vi "Analyze.vi"(0 "Analyze SHG-AK in":refnum<class "Analyze SHG-AK.lvclass">, 1 "Create Overlay?":bool, 5 "Image in":T1, 7 "Parameters":variant, 9 "Results in":variant, 11 "error in (no error)":errorcluster) -> (4 "Analyze SHG-AK out":refnum<class "Analyze SHG-AK.lvclass">, 6 "Image out":T1, 8 "Parameters out":variant, 10 "Results":variant, 15 "error out":errorcluster)   [LabVIEW 2014, in "Analyze.lvlib" / "Analyze SHG-AK.lvclass"]
uses:
  Analyze SHG-AK.lvclass
  <vilib>/vision/Image Controls.llb/IMAQ Image.ctl
  Analyze BaseClass/Analyze BaseClass.lvclass
  <vilib>/vision/NI_Vision_Development_Module.lvlib
  XDisplay/POLARIS IMAQ Display.xctl
  <vilib>/Analysis/NI_AALPro.lvlib
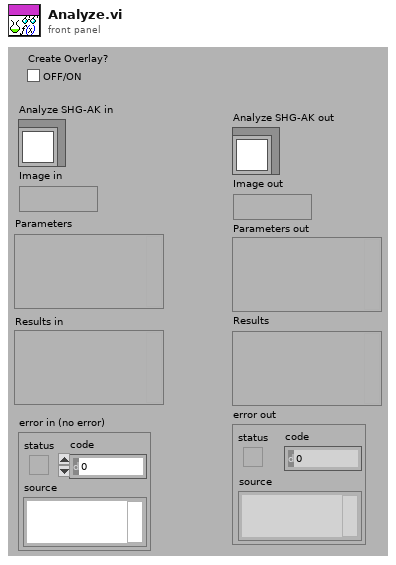
[diagram p1: front panel]
types:
  T1 = typedef "IMAQ Image.ctl" = refnum<image>
  T2 = typedef "ROI Descriptor" = cluster{"Global Rectangle":i32[], "Contours":cluster{"ID":enum32{"External", "Internal"}, "Type":u32, "Coordinates":i32[]}[]}
  T3 = cluster{"Desired Font (Application)":enum16{"User-specified Font", "Application Font", "System Font", "Dialog Font"}, "[User-specified Font]":cluster{"Font Name":string, "Size":i16, "Strikeout?":bool, "Italic?":bool, "Underline?":bool, "Outline?":bool, "Shadow?":bool, "Bold?":bool, "Rotation Angle":dbl}, "Horizontal Alignment":i16, "Vertical Alignment":i16}
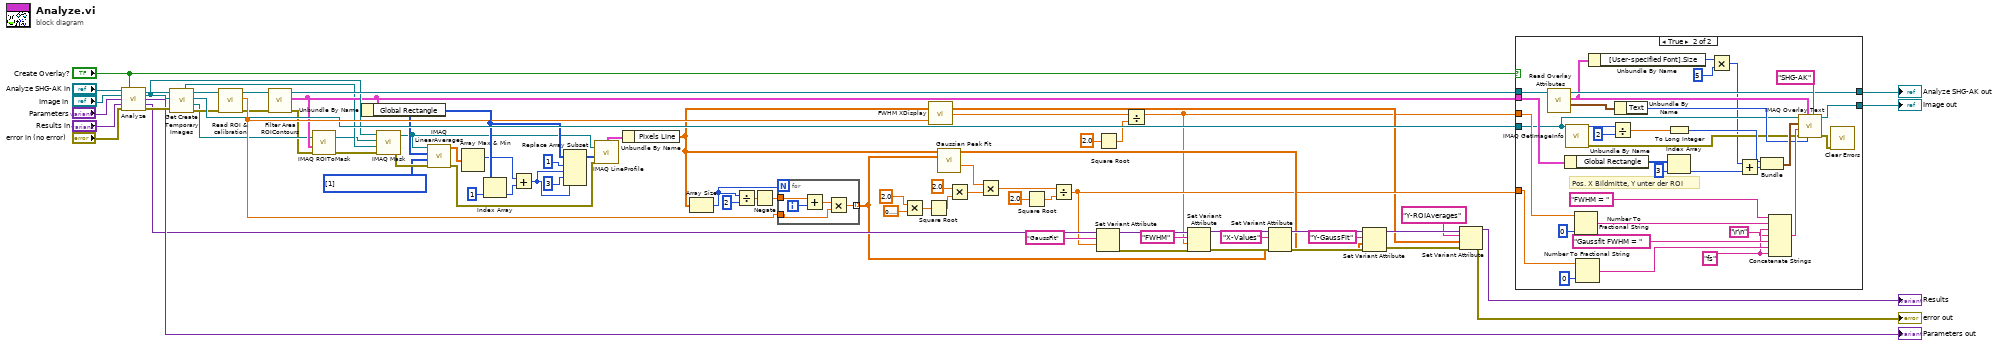
[diagram p0: block diagram]
diagram:
  w13 = i32[] [1] items=["X Axis Averages", "Y Axis Averages", "X + Y Axis Averages", "X - Y Axis Averages"] ("Averages")
  n1 = call-parent "Analyze.vi"("Analyze BaseClass in"="Analyze SHG-AK in", "Create Overlay?"="Create Overlay?", "Image in"="Image in", "Parameters"="Parameters", "Results in"="Results in", "error in (no error)"="error in (no error)") -> ("Analyze BaseClass out"=w72:refnum<class "Analyze SHG-AK.lvclass">, "Image out"=w30:T1, "Parameters out"=→"Parameters out":variant, "Results"=w54:variant, "error out"=w71:errorcluster)  [unwired: 5 in]
  n2 = call-dynamic "Get Create Temporary Images.vi"("error in (no error)"=w71, "Image in"=w30, "Analyze BaseClass in"=w72) -> ("error out"=w22:errorcluster, "image mask"=w21:T1, "work image"=w34:T1, "Analyze BaseClass out"=w23:refnum<class "Analyze SHG-AK.lvclass">, "masked image"=w20:T1)  [unwired: 4 in]
  n3 = call-dynamic "Read ROI & calibration.vi"("error in (no error)"=w22, "Analyze BaseClass in"=w23) -> ("error out"=w16:errorcluster, "calibration mm/px"=w58:dbl, "Analyze BaseClass out"=w17:refnum<class "Analyze SHG-AK.lvclass">)  [unwired: 6 in, 1 out]
  n4 = call-dynamic "Filter Area ROIContours.vi"("error in (no error)"=w16, "Analyze BaseClass in"=w17) -> ("error out"=w15:errorcluster, "ROI of Area type"=w29:T2, "Analyze BaseClass out"=w38:refnum<class "Analyze SHG-AK.lvclass">)  [unwired: 7 in]
  n5 = call "IMAQ ROIToMask"("error in (no error)"=w15, "ROI Descriptor"=w29, "Image"=w21) -> ("error out"=w19:errorcluster, "Image Out"=w18:T1)  [unwired: 3 in, 1 out]
  n6 = Unbundle By Name(w29) -> ("Global Rectangle"=w9:i32[])
  n7 = call "IMAQ Mask"("error in (no error)"=w19, "Image Dst"=w20, "Image Mask"=w18, "Image Src"=w30) -> ("error out"=w14:errorcluster, "Image Dst Out"=w4:T1)  [unwired: 1 in]
  n8 = call "IMAQ LinearAverages"("error in (no error)"=w14, "Averages"=w13, "Optional Rectangle"=w9, "Image Src"=w4) -> ("error out"=w2:errorcluster, "Y Axis Averages"=w12:sgl[])  [unwired: 3 in, 3 out]
  n9 = Array Max & Min(array=w12) -> (max index (indices)=w6:i32)  [unwired: 3 out]
  n10 = Index Array(array=w9, index=1) -> (element=w7:i32)
  n11 = Add(x=w6, y=w7) -> (x+y=w5:i32)
  n12 = Replace Array Subset(array=w9, new element #1=w5, index #1=1 ("index"), new element #2=w5, index #2=3 ("index")) -> (w3:i32[])
  n13 = call "IMAQ LineProfile"("error in (no error)"=w2, "Line Coordinates"=w3, "Image"=w4) -> ("Line Graph"=w1:cluster{"x0":sgl, "dx":sgl, "Pixels Line":sgl[]})  [unwired: 2 in, 3 out]
  n14 = Unbundle By Name(w1) -> ("Pixels Line"=w28:sgl[])
  n15 = Array Size(array=w28) -> (size(s)=w57:i32)
  n16 = Divide(x=w57, y=2) -> (x/y=w60:dbl)
  n17 = Negate(x=w60) -> (-x=w56:dbl)
  n18 = for {
    N: w57 -> [_]
    tunnel: w56 -> [w81]
    tunnel: [w79] -> w47 mode=indexing
    tunnel: w58 -> [w78]
    i -> [w82]
    n19 = Add(x=w81, y=w82) -> (x+y=w80:dbl)
    n20 = Multiply(x=w80, y=w78) -> (x*y=w79:dbl)
  }
  n21 = Multiply(x=2.0 ("y"), y=0.6931471805599453) -> (x*y=w63:dbl)
  n22 = Square Root(x=w63) -> (sqrt(x)=w64:dbl)
  n23 = call "FWHM XDisplay.vi"("calibration"=w58, "array"=w28) -> ("FHWM"=w25:dbl)
  n24 = call <vilib>:"Gaussian Peak Fit.vi"("Y"=w28, "X"=w47) -> ("Best Gaussian Fit"=w42:dbl[], "standard deviation"=w70:dbl)  [unwired: 7 in, 5 out]
  n25 = Multiply(x=2.0 ("y"), y=w64) -> (x*y=w65:dbl)
  n26 = Multiply(x=w70, y=w65) -> (x*y=w68:dbl)
  n27 = Square Root(x=2.0) -> (sqrt(x)=w67:dbl)
  n28 = Divide(x=w68, y=w67) -> (x/y=w36:dbl)
  n29 = Set Variant Attribute(Variant=w54, name="GaussFit", value=w36) -> (Variant out=w52:variant, error out=w50:errorcluster)  [unwired: 1 in, 1 out]
  n30 = Square Root(x=2.0) -> (sqrt(x)=w26:dbl)
  n31 = Divide(x=w25, y=w26) -> (x/y=w24:dbl)
  n32 = Set Variant Attribute(Variant=w52, name="FWHM", value=w24, error in=w50) -> (Variant out=w48:variant, error out=w49:errorcluster)  [unwired: 1 out]
  n33 = Set Variant Attribute(Variant=w48, name="X-Values", value=w47, error in=w49) -> (Variant out=w44:variant, error out=w45:errorcluster)  [unwired: 1 out]
  n34 = Set Variant Attribute(Variant=w44, name="Y-GaussFit", value=w42, error in=w45) -> (Variant out=w41:variant, error out=w40:errorcluster)  [unwired: 1 out]
  n35 = Set Variant Attribute(Variant=w41, name="Y-ROIAverages", value=w28, error in=w40) -> (Variant out=→"Results":variant, error out=→"error out":errorcluster)  [unwired: 1 out]
  n36 = case shown="True" "Create Overlay?" {
    tunnel: w38 -> [w84 w113]
    tunnel: w36 -> [_ w98]
    tunnel: w24 -> [_ w102]
    tunnel: [w84 w112] -> w35
    tunnel: w29 -> [_ w115]
    tunnel: w34 -> [w83 w96]
    tunnel: [w83 w95] -> w33
    frame False {
    }
    frame True {
      w87 = "fs" ("string")
      # "Pos. X Bildmitte, Y unter der ROI"
      n37 = call-dynamic "Read Overlay Attributes.vi"("Analyze BaseClass in"=w113) -> ("Overlay colors"=w111:cluster{"Border":u32, "Text":u32}, "Font, Size & Style"=w92:T3, "Analyze BaseClass out"=w112:refnum<class "Analyze SHG-AK.lvclass">)  [unwired: 6 in, 2 out]
      n38 = Unbundle By Name(w115) -> ("Global Rectangle"=w118:i32[])
      n39 = call "IMAQ GetImageInfo"("Image"=w96) -> ("error out"=w94:errorcluster, "X Resolution"=w109:i32)  [unwired: 3 in, 6 out]
      n40 = Number To Fractional String(number=w102, precision (6)=i16 0) -> (F-format string=w88:string)  [unwired: 2 in]
      n41 = Number To Fractional String(number=w98, precision (6)=i16 0) -> (F-format string=w97:string)  [unwired: 2 in]
      n42 = Unbundle By Name(w92) -> ("[User-specified Font].Size"=w90:i16)
      n43 = Divide(x=w109, y=2) -> (x/y=w107:dbl)
      n44 = Unbundle By Name(w111) -> ("Text"=w110:u32)
      n45 = To Long Integer(number=w107) -> (32bit integer=w104:i32)
      n46 = Index Array(array=w118, index=3) -> (element=w106:i32)
      n47 = Multiply(x=w90, y=i16 5) -> (x*y=w85:i16)
      n48 = Add(x=w85, y=w106) -> (x+y=w91:i32)
      n49 = Bundle(w104, w91) -> (w116:cluster{i32, i32})  [unwired: 1 in]
      n50 = Concatenate Strings("FWHM = ", w88, w87, "\r\n", "Gaussfit FWHM = ", w97, w87) -> (w117:string)
      n51 = call "IMAQ Overlay Text"("Group"="SHG-AK" ("name"), "Text Color (black)"=w110, "Font, Size & Style"=w92, "error in (no error)"=w94, "String"=w117, "Origin"=w116, "Image"=w96) -> ("error out"=w93:errorcluster, "Image Out"=w95:T1)  [unwired: 3 in]
      n52 = call <vilib>:"Clear Errors.vi"("error in (no error)"=w93) -> ()  [unwired: 5 in, 2 out]
    }
  }
  "Analyze SHG-AK out" <- w35
  "Image out" <- w33
